vi "SFC_Rep Save Repair Data.vi"(8 "error in (no error)":errorcluster caption="错误输入（无错误）", 9 "IntSerialNo":string, 10 ".NET:System.Data.DataSet":T1={"CaseSensitive"=FALSE, "Container"=refnum, "DataSetName"="", "DefaultViewManager"=refnum, "DesignMode"=FALSE, "EnforceConstraints"=FALSE, "ExtendedProperties"=refnum, "HasErrors"=FALSE, "IsInitialized"=FALSE, "Locale"=refnum, "Namespace"="", "Prefix"="", "Relations"=refnum, "RemotingFormat"=0, "SchemaSerializationMode"=1, "Site"=refnum, "Tables"=refnum} {"SchemaSerializationMode" items=["IncludeSchema"=1, "ExcludeSchema"=2]; "RemotingFormat" items=["Xml", "Binary"]}, 11 "Traceability 引用句柄":refnum<k24>) -> (0 "error out":errorcluster caption="错误输出", 2 "SFC_RepSaveRepairData":bool, 3 "Traceability 引用句柄输出":refnum<k24>)   [LabVIEW 2014, in "Traceability.lvlib"]
uses:
  Traceability.lvlib
  Traceability.dll
  System.Data
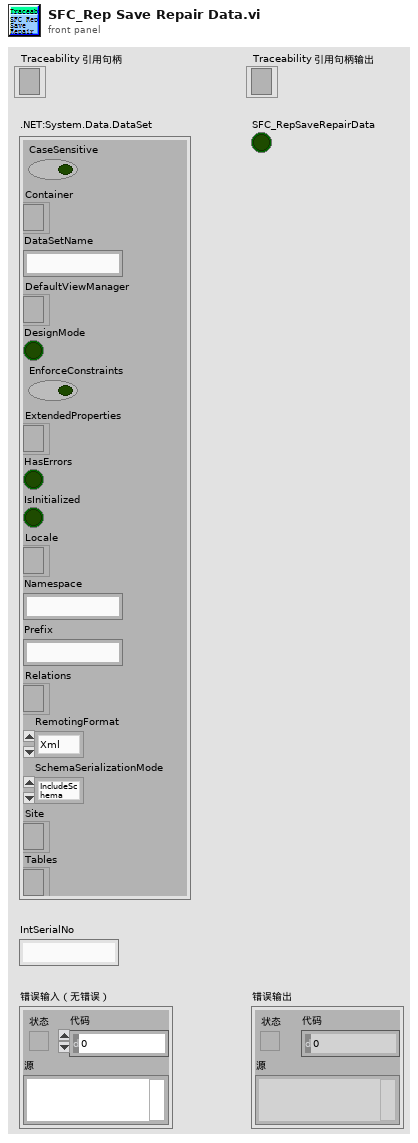
[diagram p1: front panel]
types:
  T1 = cluster{"CaseSensitive":bool, "Container":refnum<k24>, "DataSetName":string, "DefaultViewManager":refnum<k24>, "DesignMode":bool, "EnforceConstraints":bool, "ExtendedProperties":refnum<k24>, "HasErrors":bool, "IsInitialized":bool, "Locale":refnum<k24>, "Namespace":string, "Prefix":string, "Relations":refnum<k24>, "RemotingFormat":i32, "SchemaSerializationMode":i32, "Site":refnum<k24>, "Tables":refnum<k24>}
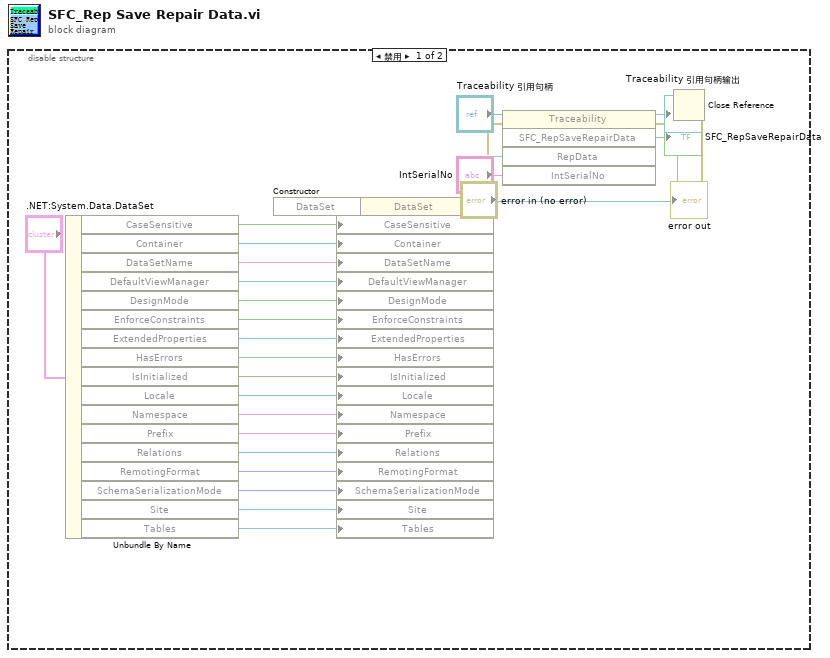
[diagram p0: block diagram]
diagram:
  n1 = disable-structure shown="禁用" {
    frame Disabled {
      n2 = Unbundle By Name(".NET:System.Data.DataSet") -> ("CaseSensitive"=w22:bool, "Container"=w21:refnum<k24>, "DataSetName"=w20:string, "DefaultViewManager"=w19:refnum<k24>, "DesignMode"=w18:bool, "EnforceConstraints"=w17:bool, "ExtendedProperties"=w16:refnum<k24>, "HasErrors"=w15:bool, "IsInitialized"=w14:bool, "Locale"=w13:refnum<k24>, "Namespace"=w12:string, "Prefix"=w11:string, "Relations"=w10:refnum<k24>, "RemotingFormat"=w9:i32, "SchemaSerializationMode"=w8:i32, "Site"=w7:refnum<k24>, "Tables"=w6:refnum<k24>)
      n3 = constructor class="DataSet"(error in="error in (no error)") -> (reference out=w26:refnum<k24>, error out=w25:errorcluster)  [unwired: 2 in, 1 out]
      n4 = property class="DataSet"(reference=w26, error in=w25, "CaseSensitive"=w22, "Container"=w21, "DataSetName"=w20, "DefaultViewManager"=w19, "DesignMode"=w18, "EnforceConstraints"=w17, "ExtendedProperties"=w16, "HasErrors"=w15, "IsInitialized"=w14, "Locale"=w13, "Namespace"=w12, "Prefix"=w11, "Relations"=w10, "RemotingFormat"=w9, "SchemaSerializationMode"=w8, "Site"=w7, "Tables"=w6) -> (reference out=w24:refnum<k24>, error out=w3:errorcluster)
      n5 = invoke class="Traceability" method="SFC_RepSaveRepairData"(reference="Traceability 引用句柄", error in=w3, "RepData"=w24, "IntSerialNo"="IntSerialNo") -> (reference out=→"Traceability 引用句柄输出":refnum<k24>, error out=w2:errorcluster, "SFC_RepSaveRepairData"=→"SFC_RepSaveRepairData":bool)  [unwired: 1 in, 2 out]
      n6 = Close Reference(reference=w24, error in (no error)=w2) -> (error out=→"error out":errorcluster)
    }
    frame Enabled {
    }
  }
